vi "Periodic Tasks.vi"(8 "error in":errorcluster) -> ()   [LabVIEW 2013]
doc: "This VI runs in parallel to other tasks. It can contain as many user-defined periodic loops as you need. These can carry out PID or other sorts of timed response."
uses:
  <vilib>/Rock Robotics/SystemInterfaces/Utilities/FPGA_UtilitiesLED Source.ctl
  <vilib>/Rock Robotics/SystemInterfaces/Utilities/FPGA_UtilitiesLED State.ctl
  <vilib>/Rock Robotics/WPI/Solenoid/WPI_SolenoidValue.ctl
  Robot Global ref.vi
  Robot Global Data.vi
  Events.vi
  <vilib>/Rock Robotics/WPI/Solenoid/WPI_SolenoidSetEnum.vi
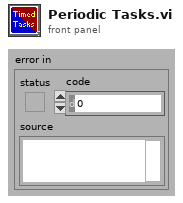
[diagram p1: front panel]
types:
  T1 = typedef "FPGA_UtilitiesLED State.ctl" = enum16{"Off", "On", "Toggle"}
  T2 = typedef "FPGA_UtilitiesLED Source.ctl" = enum16{"User LED", "FPGA LED"}
  T3 = typedef "WPI_JoystickDevRef.ctl" = cluster{"Device":T4}
  T4 = typedef "WPI_JoystickDeviceEnum.ctl" = enum16{"USB 1", "USB 2", "USB 3", "USB 4", "Kinect 1", "Kinect 2"}
  T5 = typedef "WPI_RobotDriveDevRef.ctl" = cluster{"DevStatus":errorcluster, "Motors[]":T6[], "Square Inputs":bool, "Max Output":dbl, "Isochronous":bool}
  T6 = typedef "WPI_MotorControlDeviceRef.ctl" = cluster{"DeviceStatus":errorcluster, "Type":enum16{"PWM", "CAN"}, "PWM":cluster{"Digital Module":T7, "PWM Channel":T8, "DeadBand":T9}, "CAN":cluster{"Device Number":u8, "Control Mode":T10, "Semaphore":T11, "Max Vout":dbl}, "Invert":bool, "TransformRef":T12, "InvTransformRef":T12}
  T7 = typedef "FPGA_TypedefDigitalModule.ctl" = enum16{"Digital Module 1", "Digital Module 2"}
  T8 = typedef "FPGA_DIOPWMChannel.ctl" = enum8{"PWM 1", "PWM 2", "PWM 3", "PWM 4", "PWM 5", "PWM 6", "PWM 7", "PWM 8", "PWM 9", "PWM 10", "Invalid"}
  T9 = typedef "WPI_PWMDeadband.ctl" = cluster{"Name":string, "maxPositivePwm":i32, "minPositivePwm":i32, "centerPwm":i32, "maxNegativePwm":i32, "minNegativePwm":i32, "angularRange":u16}
  T10 = typedef "WPI_CANJaguar_ControlMode.ctl" = enum8{"Percent VBus", "Current", "Speed", "Position", "Voltage"}
  T11 = typedef "Semaphore RefNum" = refnum<k1>
  T12 = typedef "WPI_PWMTransform_ConPane.ctl" = refnum<vi>
  T13 = typedef "WPI_AnalogChannelDevRef.ctl" = cluster{"DevStatus":errorcluster, "Analog Module":T14, "Analog Channel":T15}
  T14 = typedef "FPGA_TypedefAnalogModule.ctl" = enum16{"Analog Module 1", "Analog Module 2"}
  T15 = typedef "FPGA_AIChannel.ctl" = enum8{"AI 1", "AI 2", "AI 3", "AI 4", "AI 5", "AI 6", "AI 7", "AI 8", "Invalid"}
  T16 = typedef "WPI_CompressorDevRef.ctl" = cluster{"DevStatus":errorcluster, "DigitalInputDevRef":T17, "RelayDevRef":T19}
  T17 = typedef "WPI_DigitalInputDevRef.ctl" = cluster{"DevStatus":errorcluster, "DIO Channel":T18, "Digital Module":T7}
  T18 = typedef "FPGA_DIOChannel.ctl" = enum8{"DIO 1", "DIO 2", "DIO 3", "DIO 4", "DIO 5", "DIO 6", "DIO 7", "DIO 8", "DIO 9", "DIO 10", "DIO 11", "DIO 12", "DIO 13", "DIO 14", "Invalid"}
  T19 = typedef "WPI_RelayDevRef.ctl" = cluster{"DevStatus":errorcluster, "Relay Channel":T20, "Digital Module":T7, "Relay Direction":T21}
  T20 = typedef "FPGA_DIORelayChannel.ctl" = enum8{"Relay 1", "Relay 2", "Relay 3", "Relay 4", "Relay 5", "Relay 6", "Relay 7", "Relay 8", "Invalid"}
  T21 = typedef "WPI_RelayDirection.ctl" = enum16{"Both directions", "Forward only", "Reverse only"}
  T22 = typedef "WPI_SolenoidDevRef.ctl" = cluster{"DevStatus":errorcluster, "Solenoid Module":T23, "Forward Solenoid Channel":T24, "Reverse Solenoid Channel":T24}
  T23 = typedef "FPGA_TypedefSolenoidModule.ctl" = enum16{"Solenoid Module 1", "Solenoid Module 2"}
  T24 = typedef "WPI_SolenoidChannel.ctl" = enum8{"Solenoid 1", "Solenoid 2", "Solenoid 3", "Solenoid 4", "Solenoid 5", "Solenoid 6", "Solenoid 7", "Solenoid 8", "Invalid"}
  T25 = cluster{"Joysticks":cluster{"OpJoystickRef":T3, "DriveJoystickRef":T3}, "Drive Motors Ref":cluster{"RobotDriveDevRef":T5}, "Ultrasonic":cluster{"AIDeviceRef":T13}, "Comopressor":cluster{"CompressorDevRef":T16}, "Shifters":cluster{"SolenoidDevRef":T22}}
  T26 = typedef "WPI_SolenoidValue.ctl" = enum16{"Off", "On", "Forward", "Reverse"}
  T27 = cluster{"JoystickDevRef":T3, "RobotDriveDevRef":T5}
  T28 = typedef "WPI_DriverStationRobotMode2.ctl" = enum16{"Autonomous Disabled", "Autonomous Enabled", "Teleop Disabled", "Teleop Enabled", "Timeout", "Finish", "Test Disabled", "Test Enabled"}
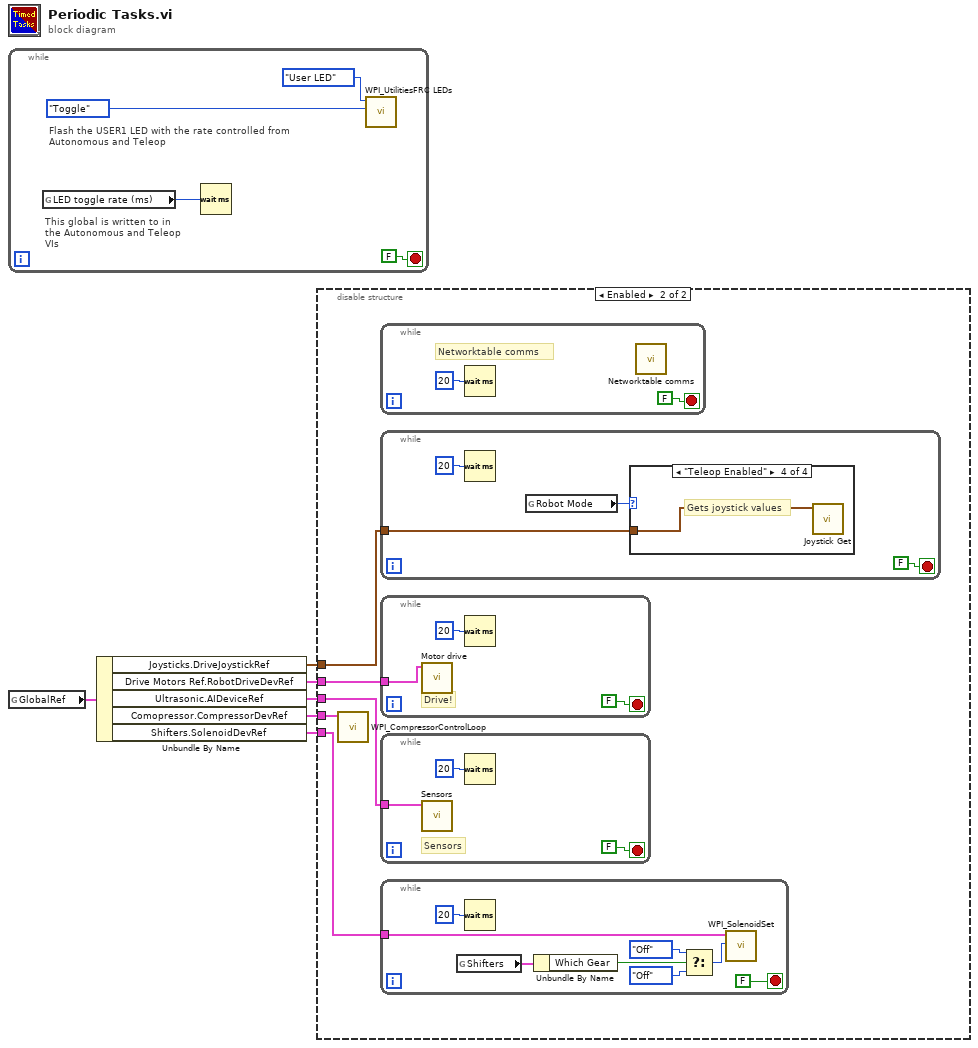
[diagram p0: block diagram]
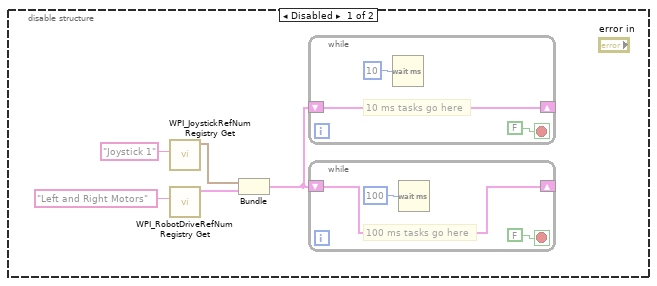
[diagram p2: hidden frame]
diagram:
  n1 = while {
    stop <- FALSE stop-if-true
    # "This global is written to in the Autonomous and Teleop VIs"
    # "Flash the USER1 LED with the rate controlled from Autonomous and Teleop"
    n2 = global read "Robot Global Data.vi" "LED toggle rate (ms)"() -> (w7:u32)
    n3 = Wait (ms)(milliseconds to wait=w7) -> ()  [unwired: 1 out]
    n4 = call <vilib>:"WPI_UtilitiesFRC LEDs.vi"("State"=FPGA_UtilitiesLED_State."Toggle", "LED Type"=FPGA_UtilitiesLED_Source."User LED") -> ()  [unwired: 1 in, 9 out]
  }
  n5 = global read "Robot Global ref.vi" "GlobalRef"() -> (w6:T25)
  n6 = Unbundle By Name(w6) -> ("Joysticks.DriveJoystickRef"=w5:T3, "Drive Motors Ref.RobotDriveDevRef"=w4:T5, "Ultrasonic.AIDeviceRef"=w3:T13, "Comopressor.CompressorDevRef"=w2:T16, "Shifters.SolenoidDevRef"=w1:T22)
  n7 = disable-structure shown="Enabled" {
    disable-tunnel: w5 -> [_ w26]
    disable-tunnel: w4 -> [_ w25]
    disable-tunnel: w3 -> [_ w24]
    disable-tunnel: w2 -> [_ w23]
    disable-tunnel: w1 -> [_ w22]
    frame Disabled {
      n8 = call <vilib>:"WPI_JoystickRefNum Registry Get.vi"("refnum name"="Joystick 1") -> ("JoystickDevRef"=w13:T3)  [unwired: 1 in, 9 out]
      n9 = call <vilib>:"WPI_RobotDriveRefNum Registry Get.vi"("refnum name"="Left and Right Motors") -> ("RobotDriveDevRef"=w12:T5)  [unwired: 1 in, 9 out]
      n10 = Bundle("JoystickDevRef"=w13, "RobotDriveDevRef"=w12) -> (w11:T27)  [unwired: 1 out]
      n11 = while {
        shift-right: [w19] -> _
        shift-left: w11 -> [w19]
        stop <- FALSE stop-if-true
        # "10 ms tasks go here"
        n12 = Wait (ms)(milliseconds to wait=u32 10) -> ()  [unwired: 1 out]
      }
      n13 = while {
        shift-right: [w16] -> _
        shift-left: w11 -> [w16]
        stop <- FALSE stop-if-true
        # "100 ms tasks go here"
        n14 = Wait (ms)(milliseconds to wait=u32 100) -> ()  [unwired: 1 out]
      }
    }
    frame Enabled {
      n15 = call <vilib>:"WPI_CompressorControlLoop.vi"("CompressorDevRef"=w23) -> ()  [unwired: 11 in]
      n16 = while {
        stop <- FALSE stop-if-true
        # "Networktable comms"
        n17 = Wait (ms)(milliseconds to wait=u32 20) -> ()  [unwired: 1 out]
        n18 = call "Networktable comms.vi"() -> ()  [unwired: 12 in]
      }
      n19 = while {
        tunnel: w26 -> [w44]
        stop <- FALSE stop-if-true
        n20 = Wait (ms)(milliseconds to wait=u32 20) -> ()  [unwired: 1 out]
        n21 = global read "Robot Global Data.vi" "Robot Mode"() -> (w46:T28)
        n22 = case shown="\"Teleop Enabled\"" w46 {
          tunnel: w44 -> [_ _ _ w47]
          frame "Autonomous Disabled", Default {
          }
          frame "Autonomous Enabled" {
          }
          frame "Teleop Disabled" {
          }
          frame "Teleop Enabled" {
            # "Gets joystick values"
            n23 = call "Joystick Get.vi"("JoystickDevRef"=w47) -> ()  [unwired: 11 in]
          }
        }
      }
      n24 = while {
        tunnel: w25 -> [w41]
        stop <- FALSE stop-if-true
        # "Drive!"
        n25 = call "Motor drive.vi"("RobotDriveDevRef"=w41) -> ()  [unwired: 11 in]
        n26 = Wait (ms)(milliseconds to wait=u32 20) -> ()  [unwired: 1 out]
      }
      n27 = while {
        tunnel: w24 -> [w37]
        stop <- FALSE stop-if-true
        # "Sensors"
        n28 = call "Sensors.vi"("Ultrasonic Sensor"=w37) -> ()  [unwired: 11 in]
        n29 = Wait (ms)(milliseconds to wait=u32 20) -> ()  [unwired: 1 out]
      }
      n30 = while {
        tunnel: w22 -> [w31]
        stop <- FALSE stop-if-true
        n31 = global read "Events.vi" "Shifters"() -> (w30:cluster{"Which Gear":bool})
        n32 = Wait (ms)(milliseconds to wait=u32 20) -> ()  [unwired: 1 out]
        n33 = Unbundle By Name(w30) -> ("Which Gear"=w29:bool)
        n34 = Select(t=WPI_SolenoidValue."Off" ("Value"), s=w29, f=WPI_SolenoidValue."Off" ("Value")) -> (s? t:f=w34:T26)
        n35 = call-poly <vilib>:"WPI_SolenoidSet.vi"("Value"=w34, "SolenoidDevRef"=w31) -> ()  [unwired: 8 in, 2 out]
      }
    }
  }
